vi "Level Array.vi"(9 "Level":u16, 10 "Min":sgl, 11 "Max":sgl) -> (3 "Level Array":sgl[](array[numeric]))   [LabVIEW 2020, in "3D Contour.lvclass"]
uses:
  <vilib>/Math Plots/3D Math Plots/3D Contour/3D Contour/3D Contour.lvclass
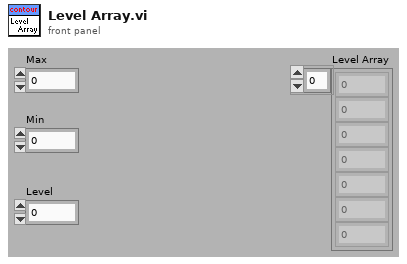
[diagram p1: front panel]
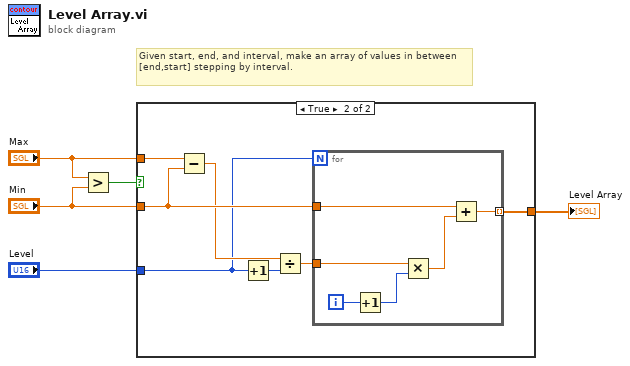
[diagram p0: block diagram]
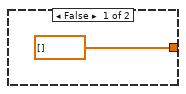
[diagram p2: hidden frame]
diagram:
  # "Given start, end, and interval, make an array of values in between [end,start] stepping by interval."
  n1 = Greater?(x="Max", y="Min") -> (0:w1:bool)
  n2 = case shown="True" w1 {
    tunnel: "Max" -> [_ w13]
    tunnel: "Level" -> [_ w8]
    tunnel: "Min" -> [_ w12]
    tunnel: [sgl[] [] w11] -> w5
    frame False {
    }
    frame True {
      n3 = Subtract(x=w13, y=w12) -> (x-y=w10:sgl)
      n4 = Increment(x=w8) -> (x+1=w7:u16)
      n5 = Divide(x=w10, y=w7) -> (x/y=w9:sgl)
      n6 = for {
        N: w8 -> [_]
        tunnel: w9 -> [w19]
        tunnel: w12 -> [w17]
        tunnel: [w16] -> w11 mode=indexing
        i -> [w15]
        n7 = Increment(x=w15) -> (x+1=w14:i32)
        n8 = Multiply(x=w19, y=w14) -> (x*y=w18:sgl)
        n9 = Add(x=w17, y=w18) -> (x+y=w16:sgl)
      }
    }
  }
  "Level Array" <- w5
